vi "Write Menu Closed Event.vi"(8 "error in (no error)":errorcluster, 10 "Menu Closed Event":refnum<user-event>, 11 "Generic Plugin in":refnum<class "Generic Plugin.lvclass">) -> (0 "error out":errorcluster, 3 "Generic Plugin out":refnum<class "Generic Plugin.lvclass">)   [LabVIEW 2011, in "Generic Plugin.lvclass"]
uses:
  Generic Plugin.lvclass
  Generic Plugin.lvclass/Generic Plugin.ctl
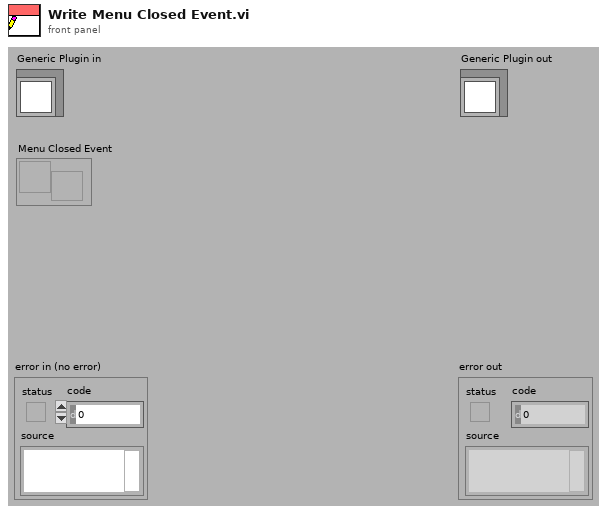
[diagram p1: front panel]
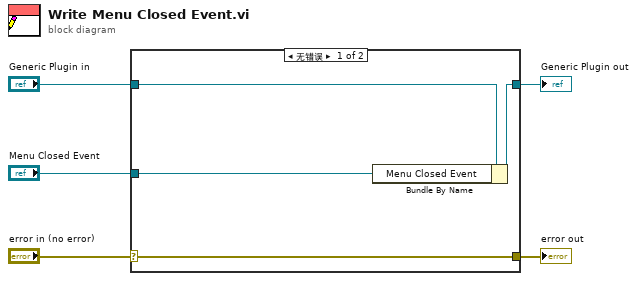
[diagram p0: block diagram]
diagram:
  n1 = case shown="无错误" "error in (no error)" {
    selector: "error in (no error)" -> [w9 w10]
    tunnel: [w9 w10] -> w4
    tunnel: [w7 w11] -> w2
    tunnel: "Generic Plugin in" -> [w8 w11]
    tunnel: "Menu Closed Event" -> [w6 _]
    frame No Error {
      n2 = Bundle By Name(cluster=w8, "Menu Closed Event"=w6) -> (w7:refnum<class "Generic Plugin.lvclass">)
    }
    frame Error {
    }
  }
  "error out" <- w4
  "Generic Plugin out" <- w2
